vi "z shm data.vi"(8 "error in (no error)":errorcluster, 11 "this_":cluster{}) -> (0 "error out":errorcluster, 3 "function return":string)   [LabVIEW 2021, in "zenohc.lvlib"]
doc: "const unsigned char *z_shm_data(const struct z_loaned_shm_t *this_);"
uses:
  zenohc.lvlib
  zenohc.dll
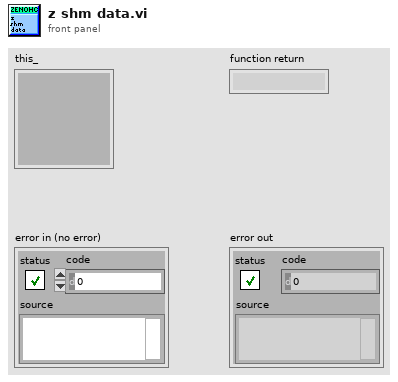
[diagram p1: front panel]
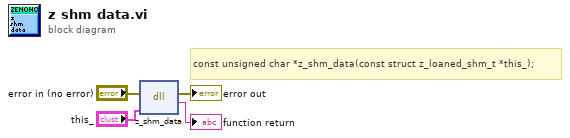
[diagram p0: block diagram]
diagram:
  # "const unsigned char *z_shm_data(const struct z_loaned_shm_t *this_);"
  n1 = dll-call lib="D:/dev/zenoh_labview/zenohc/zenohc.*" fn="z_shm_data"(error in="error in (no error)", "this_"="this_") -> (error out=→"error out":errorcluster, →"function return":string)  [unwired: 3 in, 1 out]
